vi "Flow Laser1 Trigger.vi"(1 "Delaytime(ms)":u32=200, 2 "Turn ISS Laser OFF \nand Turn Flow Laser1 ON":bool[](array[boolean])=[FALSE, TRUE, TRUE, FALSE, FALSE, FALSE, FALSE] caption="Output Data", 3 "Lines":tag="Dev1/port1/line0:1, Dev1/port1/line3:7") -> (0 "Flow Laser 1":bool)   [LabVIEW 2014]
uses:
  <vilib>/Utility/error.llb/DialogType.ctl
  <vilib>/DAQmx/create/channels.llb/DAQmx Create Channel (DO-Digital Output).vi
  <vilib>/DAQmx/write.llb/DAQmx Write (Digital 1D Bool 1Chan 1Samp).vi
panel:
  out "Flow Laser 2":bool
  # "Line    Signal\n\n0           ISS Trigger (0: OFF, 1: ON)\n1           Flow Laser 1 ON/OFF (0:OFF, 1:ON)\n2           ISS Data Acquisition (0: NO, 1: DONE)\n3           ISS Laser ON/OFF (0: ON, 1: OFF)\n4           Trigger for Marks  (0: OFF, 1: ON)\n5           Flow Laser 2 ON/OFF (0:OFF, 1:ON)\n6           Reserved\n7           Reserved"
  # "Line"
  # "0"
  # "1"
  # "3"
  # "4"
  # "5"
  # "6"
  # "7"
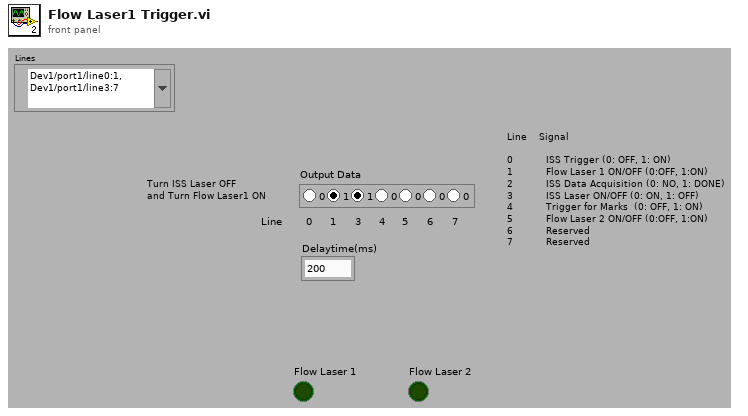
[diagram p1: front panel]
types:
  T1 = typedef "DialogType.ctl" = u16
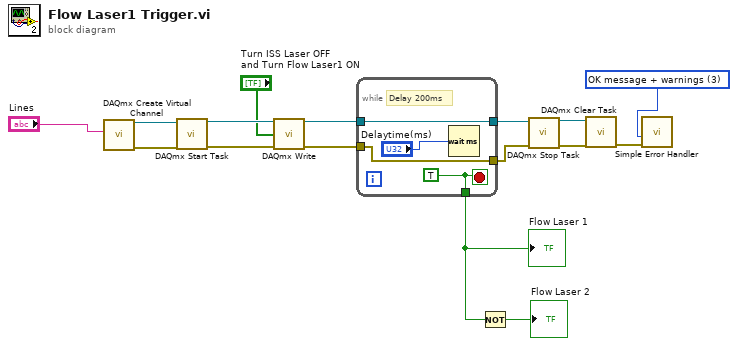
[diagram p0: block diagram]
diagram:
  w8 = T1 3 items=["no dialog", "OK message", "continue or stop message", "OK message + warnings", "continue/stop + warnings"] ("type of dialog (OK msg:1)")
  n1 = call-poly <vilib>:"DAQmx Create Virtual Channel.vi"("lines"="Lines") -> ("task out"=w11:refnum<k21>, "error out"=w10:errorcluster)  [unwired: 13 in]
  n2 = call <vilib>:"DAQmx Start Task.vi"("task/channels in"=w11, "error in"=w10) -> ("task out"=w16:refnum<k21>, "error out"=w15:errorcluster)  [unwired: 12 in]
  n3 = call-poly <vilib>:"DAQmx Write.vi"("task/channels in"=w16, "data"="Turn ISS Laser OFF \nand Turn Flow Laser1 ON", "error in"=w15) -> ("task out"=w13:refnum<k21>, "error out"=w12:errorcluster)  [unwired: 10 in, 1 out]
  n4 = while {
    tunnel: w13 -> [w20]
    tunnel: w12 -> [w19]
    tunnel: [w20] -> w5
    tunnel: [w19] -> w4
    tunnel: [w18] -> w2
    stop <- w18 stop-if-true
    w18 = TRUE
    # "Delay 200ms"
    n5 = Wait (ms)(milliseconds to wait="Delaytime(ms)") -> ()  [unwired: 1 out]
  }
  "Flow Laser 1" <- w2
  n6 = Not(x=w2) -> (.not. x?=→"Flow Laser 2":bool)
  n7 = call <vilib>:"DAQmx Stop Task.vi"("task/channels in"=w5, "error in"=w4) -> ("task out"=w7:refnum<k21>, "error out"=w6:errorcluster)  [unwired: 12 in]
  n8 = call <vilib>:"DAQmx Clear Task.vi"("task in"=w7, "error in"=w6) -> ("error out"=w9:errorcluster)  [unwired: 13 in]
  n9 = call <vilib>:"Simple Error Handler.vi"("type of dialog (OK msg:1)"=w8, "error in (no error)"=w9) -> ()  [unwired: 3 in, 5 out]
